vi "Drop (inline).vi"(6 "Copy?":bool, 7 "BetterHandle in (source)":refnum<class "BetterHandle.lvclass">, 8 "error in (no error)":errorcluster, 9 "Coords":T1, 10 "BetterDropOp":refnum<class "BetterDropOp.lvclass">, 11 "BetterHandle in (destination)":refnum<class "BetterHandle.lvclass">) -> (0 "error out":errorcluster, 3 "BetterHandle out (destination)":refnum<class "BetterHandle.lvclass">, 5 "BetterHandle out (source)":refnum<class "BetterHandle.lvclass">)   [LabVIEW 2020, in "BetterDragAndDrop.lvlib" / "BetterHandle.lvclass"]
uses:
  BetterHandle.lvclass
  BetterDropOp/BetterDropOp.lvclass
  <vilib>/Utility/miscctls.llb/LVPoint32TypeDef.ctl
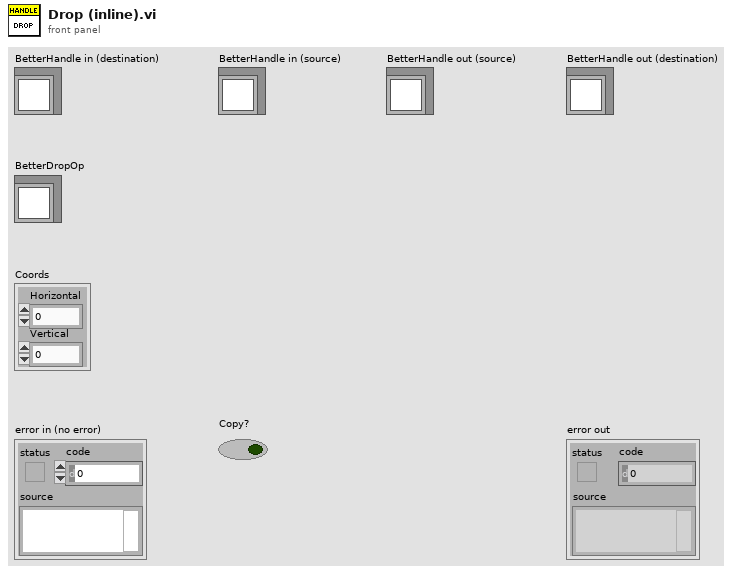
[diagram p1: front panel]
types:
  T1 = typedef "LVPoint32TypeDef.ctl" = cluster{"Horizontal":i32, "Vertical":i32}
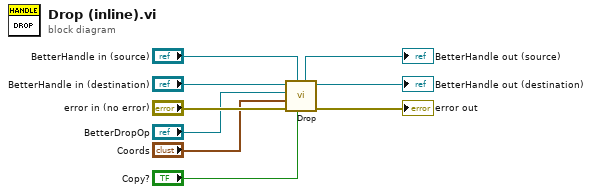
[diagram p0: block diagram]
diagram:
  n1 = call "Drop.vi"("Copy?"="Copy?", "BetterHandle in (source)"="BetterHandle in (source)", "error in (no error)"="error in (no error)", "Coords"="Coords", "BetterDropOp"="BetterDropOp", "BetterHandle in (destination)"="BetterHandle in (destination)") -> ("error out"=→"error out":errorcluster, "BetterHandle out (destination)"=→"BetterHandle out (destination)":refnum<class "BetterHandle.lvclass">, "BetterHandle out (source)"=→"BetterHandle out (source)":refnum<class "BetterHandle.lvclass">)  [unwired: 3 in]
